vi "Day 13 Task 1.vi"() -> ()   [LabVIEW 2018]
uses:
  <userlib>/_OpenG.lib/array/array.llb/Reverse 2D Array (Boolean)__ogtk.vi
panel:
  out "sum":i16
  out "result":bool[][](array[boolean])
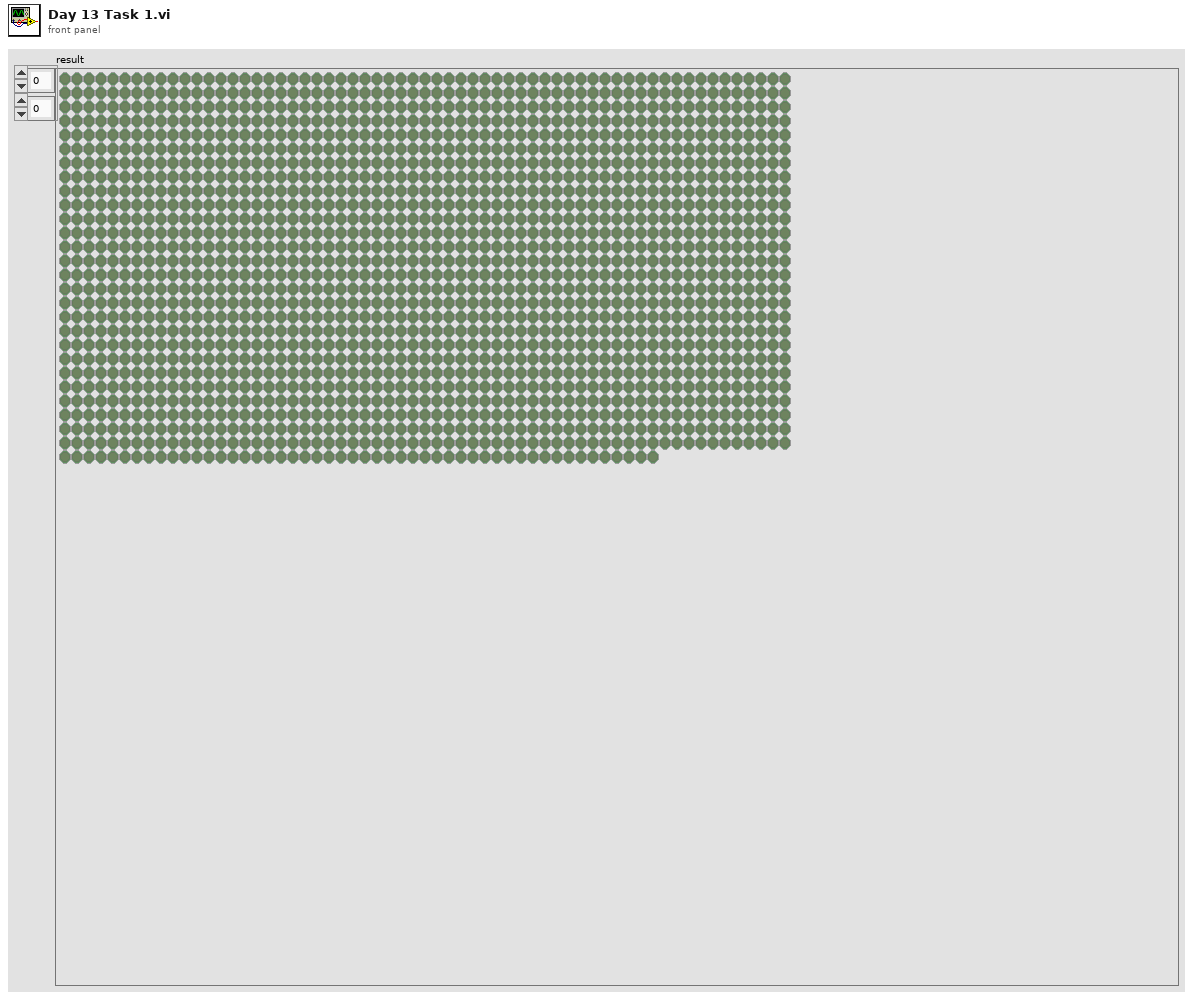
[diagram p1: front panel]
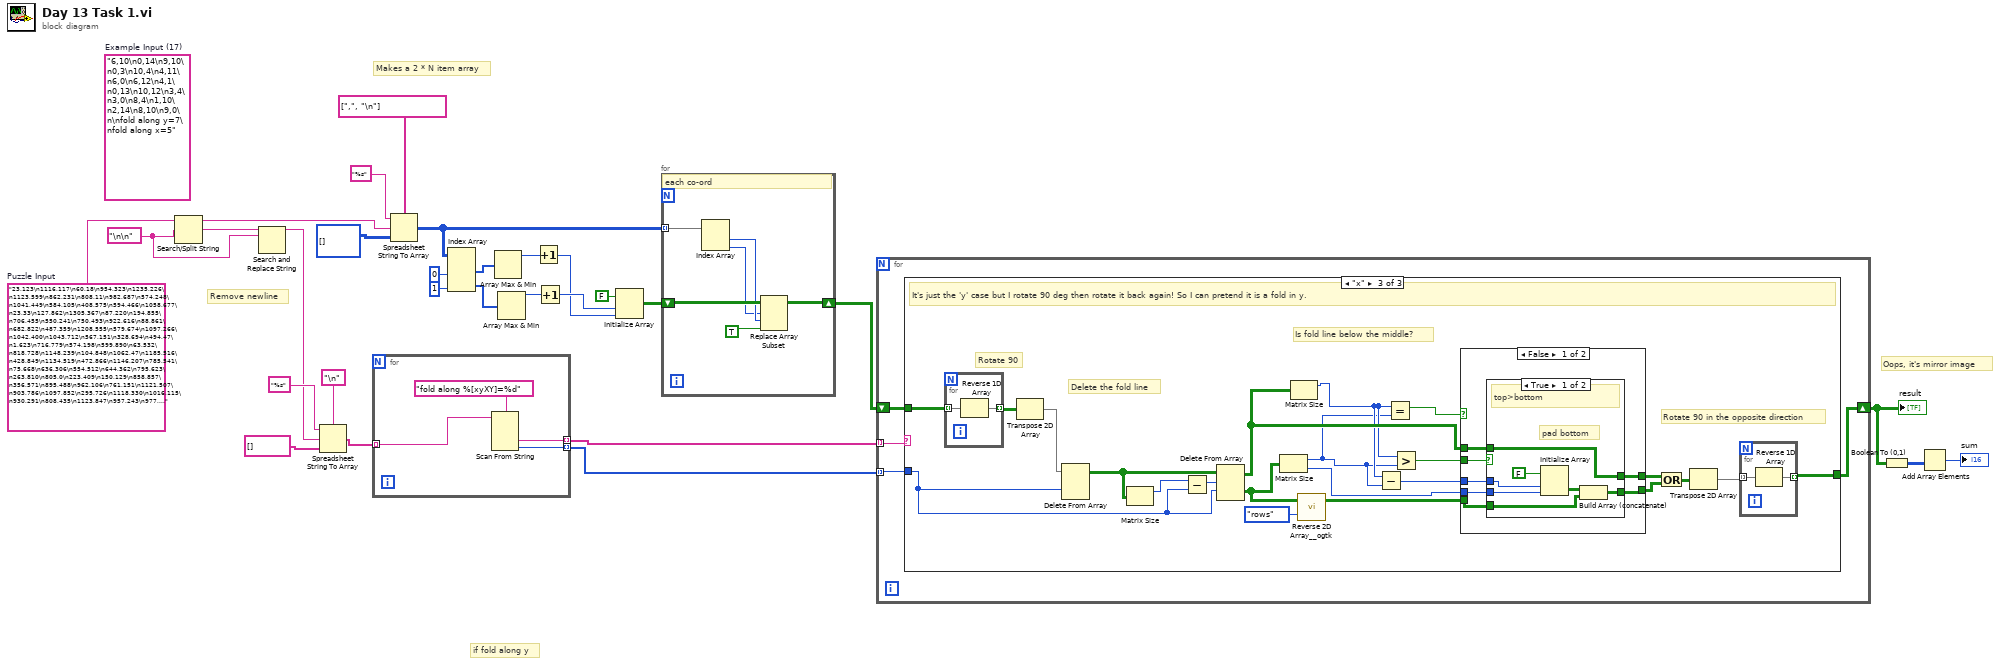
[diagram p0: block diagram]
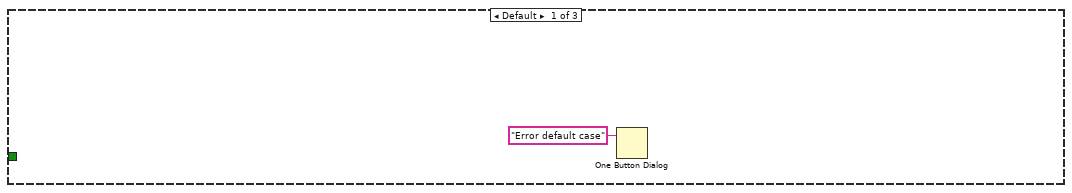
[diagram p2: hidden frame]
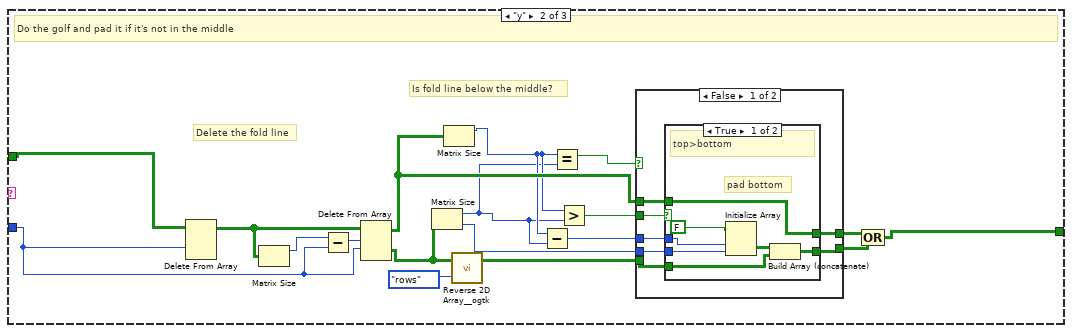
[diagram p3: hidden frame]
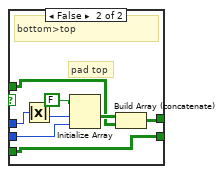
[diagram p4: hidden frame]
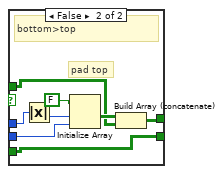
[diagram p6: hidden frame]
diagram:
  w25 = "\n\n" ("delimiter (Tab)")
  w1 = "23,123\n1116,117\n60,18\n954,323\n1235,226\n1123,599\n862,231\n808,11\n982,687\n574,248\n1041,449\n584,105\n408,575\n594,466\n1058,677\n23,33\n127,862\n1305,367\n87,220\n194,855\n706,455\n550,241\n750,493\n922,616\n88,861\n682,822\n487,359\n1208,555\n579,674\n1097,266\n1042,400\n1043,712\n567,151\n328,694\n494,47\n1,623\n716,779\n574,198\n599,890\n63,532\n818,728\n1148,239\n104,848\n1062,47\n1185,516\n428,849\n1134,519\n472,866\n1146,207\n785,541\n75,668\n636,306\n554,512\n644,362\n795,623\n263,810\n805,0\n223,409\n150,129\n858,857\n356,571\n895,488\n962,106\n761,151\n1121,507\n903,786\n1097,852\n295,726\n1118,330\n1016,115\n930,291\n808,435\n1123,847\n957,243\n977,371\n492,207\n654,229\n1285,401\n560,401\n94,65\n1110,110\n492,840\n922,242\n798,248\n252,257\n333,819\n410,855\n1218,800\n157,582\n176,519\n1001,390\n843,599\n572,185\n875,9\n383,697\n310,369\n731,220\n770,600\n638,861\n284,599\n950,779\n927,4\n949,729\n493,712\n105,66\n989,527\n68,65\n743,743\n862,103\n681,744\n855,32\n216,519\n1054,592\n551,854\n482,651\n1009,651\n408,319\n967,596\n276,23\n898,819\n654,205\n88,413\n353,722\n1263,407\n1140,553\n1228,864\n435,697\n763,505\n817,182\n301,620\n67,203\n448,663\n575,254\n736,78\n378,103\n154,427\n858,37\n852,628\n1228,870\n113,714\n929,523\n68,737\n212,250\n893,343\n438,71\n713,439\n636,361\n624,599\n31,714\n579,519\n346,533\n830,429\n718,142\n817,574\n1048,145\n430,71\n930,689\n161,320\n689,486\n346,197\n75,226\n1103,376\n114,294\n26,854\n912,302\n452,185\n870,327\n152,429\n1128,890\n711,645\n509,35\n170,553\n326,687\n1004,788\n92,773\n907,488\n94,493\n825,683\n823,298\n296,74\n565,343\n1225,837\n746,763\n566,497\n719,138\n674,140\n565,791\n1031,25\n756,382\n572,750\n970,312\n661,527\n478,631\n385,445\n940,599\n343,596\n490,217\n242,371\n266,779\n267,485\n437,259\n984,709\n957,401\n908,257\n1208,339\n472,25\n1148,207\n80,528\n602,155\n256,766\n300,822\n266,331\n703,745\n1196,824\n657,271\n105,599\n612,373\n594,690\n25,172\n750,829\n442,376\n1153,582\n741,389\n818,168\n120,103\n105,295\n497,312\n395,467\n274,801\n672,33\n497,582\n1200,179\n378,455\n855,862\n1197,714\n1059,889\n698,344\n472,28\n1016,779\n597,147\n899,304\n395,469\n306,340\n1310,431\n1146,640\n1074,315\n500,427\n108,166\n959,175\n1240,302\n1260,730\n1016,180\n1221,103\n846,70\n480,569\n161,350\n440,567\n199,338\n1160,71\n1098,518\n410,487\n922,278\n80,590\n1284,854\n518,182\n448,215\n818,743\n370,295\n657,719\n1020,84\n1193,703\n604,791\n55,249\n801,511\n1093,784\n813,771\n1089,887\n1052,487\n920,736\n176,263\n1246,525\n460,295\n226,493\n872,715\n820,239\n761,131\n739,182\n556,329\n1235,648\n437,612\n815,410\n160,847\n1292,82\n1235,668\n1178,599\n892,763\n343,148\n738,127\n1061,249\n935,645\n433,887\n1131,746\n925,893\n873,730\n194,151\n1136,17\n200,784\n744,145\n607,697\n1240,105\n686,329\n244,870\n700,586\n575,640\n1109,49\n1016,107\n518,614\n724,65\n800,138\n224,823\n952,341\n1230,366\n410,821\n455,191\n1168,218\n1016,787\n206,7\n922,204\n120,93\n70,275\n382,504\n247,152\n571,712\n1150,651\n1098,376\n92,121\n520,11\n766,295\n161,847\n731,648\n674,533\n1173,59\n1206,166\n75,815\n838,28\n547,284\n1059,375\n873,110\n865,639\n982,709\n213,852\n1044,375\n1149,126\n333,371\n1149,847\n790,235\n790,424\n1148,280\n430,451\n492,743\n798,218\n930,205\n706,791\n1039,4\n1230,360\n1066,463\n301,651\n1068,819\n594,39\n1066,487\n567,562\n202,37\n649,771\n147,298\n1001,607\n370,599\n1218,773\n654,431\n5,571\n32,474\n649,99\n596,877\n1156,427\n1305,323\n694,261\n1228,30\n634,19\n87,444\n360,740\n291,423\n1150,847\n5,435\n199,556\n1014,74\n300,166\n879,409\n18,809\n266,107\n796,848\n1228,278\n810,651\n1148,640\n689,802\n857,180\n251,599\n1151,87\n403,406\n1205,831\n358,341\n30,372\n795,271\n775,824\n1223,599\n279,25\n1255,249\n907,182\n1208,4\n1059,22\n251,630\n515,795\n817,798\n748,374\n80,78\n162,726\n402,257\n68,267\n1292,361\n142,676\n1248,528\n120,175\n190,376\n676,19\n470,646\n32,698\n1263,597\n502,667\n1149,544\n488,495\n1134,631\n1128,442\n1294,481\n102,339\n403,712\n756,512\n1205,105\n1034,455\n698,550\n878,196\n1059,630\n1253,455\n709,707\n328,872\n1146,616\n795,520\n498,161\n492,54\n1064,870\n388,876\n306,788\n83,182\n852,644\n1243,649\n962,340\n713,893\n631,439\n837,623\n314,312\n1094,519\n1120,518\n540,152\n957,722\n145,35\n1230,590\n353,493\n564,539\n1310,17\n1134,263\n1171,679\n801,859\n679,571\n390,736\n30,522\n1222,481\n346,362\n110,715\n556,565\n739,712\n932,775\n818,463\n813,562\n351,271\n760,512\n930,603\n1009,620\n875,197\n294,107\n800,756\n761,295\n754,117\n985,240\n843,123\n430,823\n1183,862\n596,46\n873,612\n1173,271\n49,42\n1190,175\n575,780\n1252,877\n493,126\n246,814\n370,792\n636,140\n888,513\n668,877\n1168,676\n1278,698\n1039,325\n515,495\n353,274\n736,304\n801,280\n67,691\n1173,835\n552,787\n417,343\n1208,611\n503,366\n1066,95\n1285,72\n1128,4\n547,616\n380,205\n62,116\n952,820\n656,431\n218,215\n716,428\n741,421\n1034,23\n125,516\n1248,401\n1261,852\n540,742\n422,381\n161,544\n395,427\n1044,204\n268,429\n900,407\n465,620\n989,819\n1298,358\n266,519\n1138,651\n607,197\n1158,883\n452,37\n110,599\n518,56\n713,455\n1033,614\n1160,765\n990,301\n982,648\n877,763\n251,648\n845,835\n638,481\n277,614\n525,353\n880,778\n385,595\n1247,810\n629,296\n351,207\n967,148\n1021,845\n1287,123\n1230,78\n1309,623\n378,775\n445,703\n85,841\n1015,714\n328,246\n1240,773\n838,4\n908,665\n686,388\n996,312\n843,151\n264,158\n714,46\n308,85\n412,819\n957,493\n1059,246\n377,311\n1026,102\n711,281\n1203,389\n925,445\n353,401\n893,327\n610,819\n52,801\n259,467\n388,564\n1197,628\n100,717\n950,714\n893,567\n266,375\n668,536\n127,639\n808,465\n744,397\n852,451\n55,4\n818,239\n892,131\n1009,274\n855,480\n518,824\n1223,295\n33,817\n822,495\n977,523\n1002,697\n748,520\n1290,467\n25,822\n251,246\n1041,893\n1059,488\n161,768\n816,847\n249,249\n880,823\n408,304\n388,690\n1248,569\n594,652\n16,481\n1305,459\n74,677\n136,166\n119,518\n623,180\n458,266\n251,519\n388,151\n708,801\n951,266\n1196,294\n177,336\n1158,459\n1160,317\n1191,471\n296,777\n1098,250\n1063,742\n703,597\n1101,221\n612,344\n1190,353\n679,439\n892,315\n1272,485\n850,295\n64,369\n872,519\n293,481\n535,423\n852,3\n838,866\n1036,291\n902,192\n1004,340\n656,229\n258,407\n201,845\n50,455\n1231,192\n714,848\n330,502\n60,428\n137,274\n381,355\n94,519\n838,476\n1178,71\n761,383\n584,789\n246,575\n982,694\n437,784\n489,488\n1235,465\n1228,37\n679,887\n1044,71\n895,854\n1103,518\n855,191\n718,752\n1212,677\n549,579\n162,239\n1279,180\n584,856\n1190,599\n1059,599\n544,715\n890,542\n1150,47\n862,64\n246,870\n1064,360\n586,737\n922,330\n1230,95\n673,831\n1000,77\n55,697\n731,519\n928,390\n624,372\n1087,409\n616,485\n1101,255\n189,620\n1019,526\n1174,182\n562,374\n549,131\n403,488\n403,441\n152,883\n169,582\n1223,220\n952,74\n607,297\n187,599\n251,872\n621,408\n433,7\n939,87\n85,837\n102,283\n689,856\n82,864\n801,35\n566,749\n410,521\n259,873\n1093,612\n344,677\n364,810\n85,57\n1088,205\n1247,362\n75,648\n705,42\n156,553\n139,99\n808,429\n247,332\n817,768\n902,543\n873,259\n684,771\n502,435\n850,487\n1235,815\n716,652\n64,525\n120,295\n1173,274\n574,534\n1140,789\n525,541\n1230,304\n92,374\n1285,722\n113,628\n277,280\n888,401\n688,628\n330,392\n12,877\n402,637\n216,375\n852,266\n903,376\n838,869\n1205,63\n1064,319\n817,350\n177,560\n877,7\n1280,295\n890,32\n510,866\n408,360\n433,763\n764,679\n75,79\n221,828\n410,463\n1174,630\n954,123\n28,571\n740,814\n587,691\n1206,868\n217,784\n621,861\n602,603\n1212,217\n120,541\n432,196\n382,390\n915,469\n67,649\n959,719\n82,687\n502,121\n1242,65\n514,848\n1160,711\n862,887\n653,271\n1218,374\n152,569\n681,296\n957,274\n810,427\n473,271\n411,590\n649,123\n294,180\n982,872\n221,66\n271,773\n550,512\n766,179\n546,215\n159,484\n432,56\n321,527\n689,408\n748,800\n348,106\n70,302\n478,183\n656,241\n458,331\n246,80\n276,455\n1026,743\n1250,18\n62,528\n964,197\n340,582\n266,115\n49,852\n575,562\n206,887\n223,485\n1278,180\n218,231\n107,697\n724,157\n989,371\n908,637\n1242,829\n32,180\n922,652\n738,750\n137,59\n751,245\n875,726\n82,633\n112,7\n\nfold along x=655\nfold along y=447\nfold along x=327\nfold along y=223\nfold along x=163\nfold along y=111\nfold along x=81\nfold along y=55\nfold along x=40\nfold along y=27\nfold along y=13\nfold along y=6"  # Puzzle Input
  (unwired) "6,10\n0,14\n9,10\n0,3\n10,4\n4,11\n6,0\n6,12\n4,1\n0,13\n10,12\n3,4\n3,0\n8,4\n1,10\n2,14\n8,10\n9,0\n\nfold along y=7\nfold along x=5"  # Example Input (17)
  # "Oops, it's mirror image"
  # "if fold along y"
  # "Remove newline"
  # "Makes a 2 * N item array"
  n1 = Search/Split String(string=w1, search string/char (-)=w25) -> (substring before match=w24:string, match + rest of string=w26:string)  [unwired: 1 in, 1 out]
  n2 = Search and Replace String(input string=w26, search string=w25) -> (result string=w8:string)  [unwired: 6 in, 3 out]
  n3 = Spreadsheet String To Array(delimiter (Tab)="\n", format string="%s", spreadsheet string=w8, array type (2D Dbl)=string[] []) -> (array=w9:string[])
  n4 = for {
    tunnel: w9 -> [w32] mode=indexing
    tunnel: [w31] -> w3 mode=indexing
    tunnel: [w30] -> w2 mode=indexing
    n5 = Scan From String(format string="fold along %[xyXY]=%d", input string=w32) -> (output 1=w31:string, output 2=w30:i32)  [unwired: 4 in, 3 out]
  }
  n6 = Spreadsheet String To Array(delimiter (Tab)=string[] [",", "\n"], format string="%s", spreadsheet string=w24, array type (2D Dbl)=i32[][] []) -> (array=w23:i32[][])
  n7 = Index Array(array=w23, index (col) #1=0 ("disabled index (col)"), index (col) #2=1 ("index (col)")) -> (element #1=w20:i32[], element #2=w19:i32[])  [unwired: 2 in]
  n8 = Array Max & Min(array=w20) -> (max value=w16:i32)  [unwired: 3 out]
  n9 = Array Max & Min(array=w19) -> (max value=w15:i32)  [unwired: 3 out]
  n10 = Increment(x=w16) -> (x+1=w13:i32)
  n11 = Increment(x=w15) -> (x+1=w14:i32)
  n12 = Initialize Array(FALSE, w14, w13) -> (w17:bool[][])
  n13 = for {
    tunnel: w23 -> [w37] mode=indexing
    shift-right: [w38] -> w4
    shift-left: w17 -> [w39]
    # "each co-ord"
    n14 = Index Array(array=w37) -> (element #1=w36:i32, element #2=w35:i32)  [unwired: 2 in]
    n15 = Replace Array Subset(array=w39, new element=TRUE, index (row)=w35, index (col)=w36) -> (w38:bool[][])
  }
  n16 = for {
    tunnel: w2 -> [w41] mode=indexing
    tunnel: w3 -> [w42] mode=indexing
    shift-right: [w40] -> w7
    shift-left: w4 -> [w43]
    n17 = case shown="\"x\"" w42 {
      tunnel: w43 -> [_ w61 w92]
      tunnel: w41 -> [_ w57 w90]
      tunnel: [_ w45 w87] -> w40
      frame Default {
        n18 = One Button Dialog(message="Error default case") -> ()  [unwired: 1 in, 1 out]
      }
      frame "y" {
        # "Is fold line below the middle?"
        # "Delete the fold line"
        # "Do the golf and pad it if it's not in the middle"
        n19 = Delete From Array(array=w61, index (row)=w57) -> (array with subset deleted=w60:bool[][])  [unwired: 2 in, 1 out]
        n20 = Matrix Size(0:w60) -> (1:w58:i32)  [unwired: 1 out]
        n21 = Subtract(x=w58, y=w57) -> (x-y=w59:i32)
        n22 = Delete From Array(array=w60, length=w59, index (row)=w57) -> (deleted portion=w56:bool[][], array with subset deleted=w52:bool[][])  [unwired: 1 in]
        n23 = Matrix Size(0:w56) -> (1:w48:i32, 2:w50:i32)
        n24 = Matrix Size(0:w52) -> (1:w49:i32)  [unwired: 1 out]
        n25 = call-poly <userlib>:"Reverse 2D Array__ogtk.vi"("by rows or columns (rows)"=enum16{"rows", "columns"}."rows", "Array"=w56) -> ("Reversed Array"=w53:bool[][])  [unwired: 1 in]
        n26 = Subtract(x=w49, y=w48) -> (x-y=w47:i32)
        n27 = Equal?(x=w49, y=w48) -> (x = y?=w55:bool)
        n28 = Greater?(x=w49, y=w48) -> (0:w46:bool)
        n29 = case shown="False" w55 {
          tunnel: [w66 w86] -> w54
          tunnel: w53 -> [w67 w86]
          tunnel: w52 -> [w63 w85]
          tunnel: [w64 w85] -> w51
          tunnel: w50 -> [w69 _]
          tunnel: w47 -> [w68 _]
          tunnel: w46 -> [w65 _]
          frame False {
            n30 = case shown="True" w65 {
              tunnel: w69 -> [w76 w84]
              tunnel: w68 -> [w75 w82]
              tunnel: w67 -> [w72 w77]
              tunnel: [w71 w77] -> w66
              tunnel: [w70 w80] -> w64
              tunnel: w63 -> [w70 w78]
              frame True {
                # "pad bottom"
                # "top>bottom"
                n31 = Initialize Array(FALSE, w75, w76) -> (w74:bool[][])
                n32 = Build Array (concatenate)(w74, w72) -> (w71:bool[][])
              }
              frame False {
                # "pad top"
                # "bottom>top"
                n33 = Absolute Value(x=w82) -> (abs(x)=w81:i32)
                n34 = Initialize Array(FALSE, w81, w84) -> (w79:bool[][])
                n35 = Build Array (concatenate)(w79, w78) -> (w80:bool[][])
              }
            }
          }
          frame True {
            # "Do nothing"
          }
        }
        n36 = Compound Arithmetic op=OR(w51, w54) -> (w45:bool[][])
      }
      frame "x" {
        # "Rotate 90 in the opposite direction"
        # "Rotate 90"
        # "Is fold line below the middle?"
        # "Delete the fold line"
        # "It's just the 'y' case but I rotate 90 deg then rotate it back again! So I can pretend it is a fold in y."
        n37 = for {
          tunnel: w92 -> [w112] mode=indexing
          tunnel: [w111] -> w93 mode=indexing
          n38 = Reverse 1D Array(array=w112) -> (reversed array=w111:bool[])
        }
        n39 = Transpose 2D Array(2D array=w93) -> (transposed array=w91:bool[][])
        n40 = Delete From Array(array=w91, index (row)=w90) -> (array with subset deleted=w107:bool[][])  [unwired: 2 in, 1 out]
        n41 = Matrix Size(0:w107) -> (1:w105:i32)  [unwired: 1 out]
        n42 = Subtract(x=w105, y=w90) -> (x-y=w106:i32)
        n43 = Delete From Array(array=w107, length=w106, index (row)=w90) -> (deleted portion=w104:bool[][], array with subset deleted=w101:bool[][])  [unwired: 1 in]
        n44 = Matrix Size(0:w104) -> (1:w97:i32, 2:w99:i32)
        n45 = Matrix Size(0:w101) -> (1:w98:i32)  [unwired: 1 out]
        n46 = call-poly <userlib>:"Reverse 2D Array__ogtk.vi"("by rows or columns (rows)"=enum16{"rows", "columns"}."rows", "Array"=w104) -> ("Reversed Array"=w102:bool[][])  [unwired: 1 in]
        n47 = Subtract(x=w98, y=w97) -> (x-y=w96:i32)
        n48 = Equal?(x=w98, y=w97) -> (x = y?=w103:bool)
        n49 = Greater?(x=w98, y=w97) -> (0:w95:bool)
        n50 = case shown="False" w103 {
          tunnel: [w116 w136] -> w94
          tunnel: w102 -> [w117 w136]
          tunnel: w101 -> [w113 w135]
          tunnel: [w114 w135] -> w100
          tunnel: w99 -> [w119 _]
          tunnel: w96 -> [w118 _]
          tunnel: w95 -> [w115 _]
          frame False {
            n51 = case shown="True" w115 {
              tunnel: w119 -> [w126 w134]
              tunnel: w118 -> [w125 w132]
              tunnel: w117 -> [w122 w127]
              tunnel: [w121 w127] -> w116
              tunnel: [w120 w130] -> w114
              tunnel: w113 -> [w120 w128]
              frame True {
                # "pad bottom"
                # "top>bottom"
                n52 = Initialize Array(FALSE, w125, w126) -> (w124:bool[][])
                n53 = Build Array (concatenate)(w124, w122) -> (w121:bool[][])
              }
              frame False {
                # "pad top"
                # "bottom>top"
                n54 = Absolute Value(x=w132) -> (abs(x)=w131:i32)
                n55 = Initialize Array(FALSE, w131, w134) -> (w129:bool[][])
                n56 = Build Array (concatenate)(w129, w128) -> (w130:bool[][])
              }
            }
          }
          frame True {
            # "Do nothing"
          }
        }
        n57 = Compound Arithmetic op=OR(w100, w94) -> (w89:bool[][])
        n58 = Transpose 2D Array(2D array=w89) -> (transposed array=w88:bool[][])
        n59 = for {
          tunnel: w88 -> [w110] mode=indexing
          tunnel: [w109] -> w87 mode=indexing
          n60 = Reverse 1D Array(array=w110) -> (reversed array=w109:bool[])
        }
      }
    }
  }
  "result" <- w7
  n61 = Boolean To (0,1)(Boolean=w7) -> (0, 1=w6:i16[][])
  n62 = Add Array Elements(numeric array=w6) -> (sum=→"sum":i16)
